vi "Untitled 1 (SubVI).vi"(4 "L0":i32, 6 "L1":i32, 9 "Y1":i32, 10 "X1":i32) -> (7 "theta 0":i32, 8 "theta 1":i32)   [LabVIEW 2014]
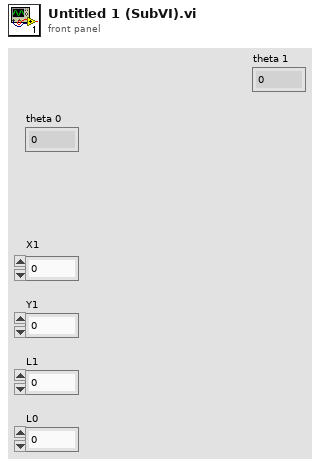
[diagram p1: front panel]
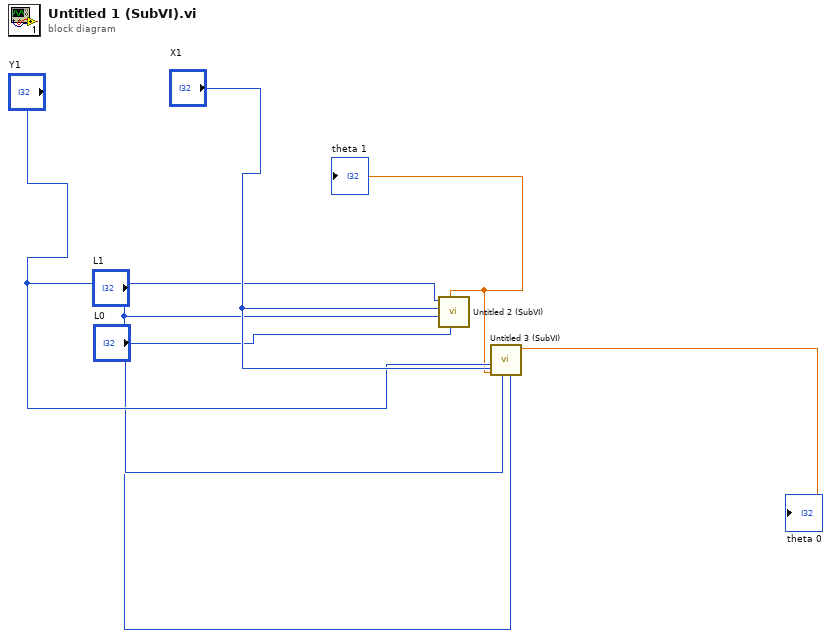
[diagram p0: block diagram]
diagram:
  n1 = call "Untitled 2 (SubVI).vi"("L0"="L0", "L1"="L1", "X"="X1", "Y"="Y1") -> ("Numeric"=w1:dbl)  [unwired: 7 in]
  "theta 1" <- w1
  n2 = call "Untitled 3 (SubVI).vi"("L1"="L1", "X"="X1", "L0"="L0", "theta 1"=w1, "Y"="Y1") -> ("theta 0"=→"theta 0":dbl)  [unwired: 6 in]
